vi "Format Monitor_State_LVXML.vi"(1 "xmlData in":T2, 3 "error in (no error)":errorcluster) -> (8 "Value":string, 10 "error out":errorcluster)   [LabVIEW 2014, in "AWS_EC2.lvlib" / "AWS_EC2.lvclass"]
uses:
  AWS_EC2.lvclass
  lv-xml-parser/r0/trunk/VI Source/EventType.ctl
  lv-xml-parser/r0/trunk/VI Source/LV XML Parser.lvlib
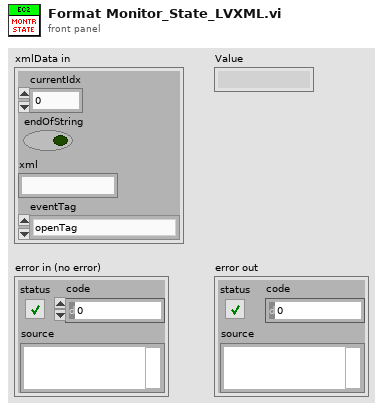
[diagram p1: front panel]
types:
  T1 = typedef "LV XML Parser.lvlib/EventType.ctl" = enum16{"openTag", "endOpenTag", "closeTag", "comment", "endComment", "endOfFile", "attribute", "startXml"}
  T2 = cluster{"currentIdx":i32, "endOfString":bool, "xml":string, "eventTag":T1}
  T3 = cluster{"namespaceUri":string, "localName":string}
  T4 = cluster{"Attributes":cluster{"localName":string, "namespaceUri":string, "value":string}[], "localName":string, "namespaceUri":string, "valueXmlData":cluster{"currentIdx":i32, "endOfString":bool, "xml":string, "eventTag":T1}}[]
  T5 = cluster{"Attributes":cluster{"localName":string, "namespaceUri":string, "value":string}[], "localName":string, "namespaceUri":string, "valueXmlData":cluster{"currentIdx":i32, "endOfString":bool, "xml":string, "eventTag":T1}}
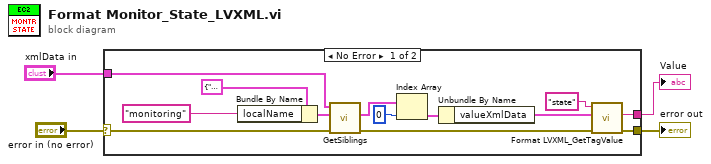
[diagram p0: block diagram]
diagram:
  n1 = case shown="No Error" "error in (no error)" {
    selector: "error in (no error)" -> [w5 w18]
    tunnel: "xmlData in" -> [w8 _]
    tunnel: [w7 _] -> w3
    tunnel: [w6 w18] -> w4
    frame No Error {
      n2 = Bundle By Name(cluster=T3 {"namespaceUri"="", "localName"=""} ("limitToTag"), "localName"="monitoring" ("Tag name")) -> (w16:T3)
      n3 = call "GetSiblings.vi"("error in (no error)"=w5, "limitToTag"=w16, "xmlData"=w8) -> ("error out"=w10:errorcluster, "Siblings"=w13:T4)  [unwired: 7 in]
      n4 = Index Array(array=w13, index=0) -> (element=w11:T5)
      n5 = Unbundle By Name(w11) -> ("valueXmlData"=w12:T2)
      n6 = call "Format LVXML_GetTagValue.vi"("error in (no error)"=w10, "xmlDataIn"=w12, "Tag name"="state") -> ("error out"=w6:errorcluster, "Value"=w7:string)  [unwired: 6 in, 1 out]
    }
    frame Error {
    }
  }
  "error out" <- w4
  "Value" <- w3
